vi "C37 DLL Shutdown.vi"(8 "error in (no error)":errorcluster) -> (0 "error out":errorcluster)   [LabVIEW 2018, in "S3DK.lvlib" / "C37118-DLL.lvlib"]
uses:
  C37118-DLL.lvlib
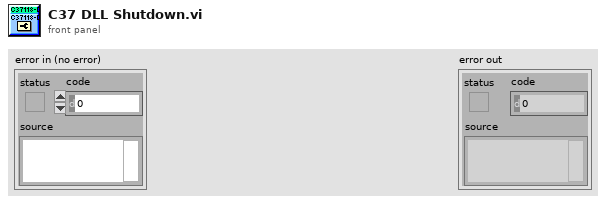
[diagram p1: front panel]
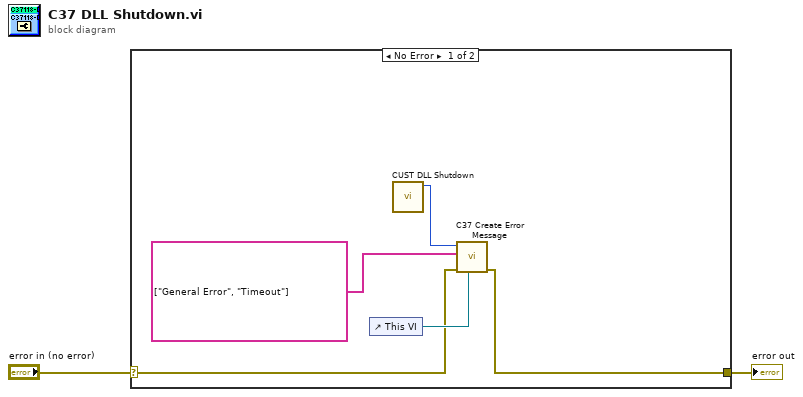
[diagram p0: block diagram]
diagram:
  n1 = case shown="No Error" "error in (no error)" {
    selector: "error in (no error)" -> [w6 w8]
    tunnel: [w5 w8] -> w2
    frame No Error {
      n2 = control-ref of="This VI"() -> (w7:refnum<vi>)
      n3 = call "CUST DLL Shutdown.vi"() -> ("function return"=w3:i32)  [unwired: 11 in]
      n4 = call "C37 Create Error Message.vi"("VI Reference"=w7, "error in (no error)"=w6, "Error Messages"=string[] ["General Error", "Timeout"], "function return"=w3) -> ("error out"=w5:errorcluster)  [unwired: 7 in]
    }
    frame Error {
    }
  }
  "error out" <- w2
